vi "Set Z Voltage_test.vi"(2 "Z-Position":dbl) -> ()   [LabVIEW 2014]
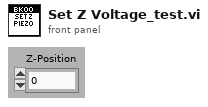
[diagram p1: front panel]
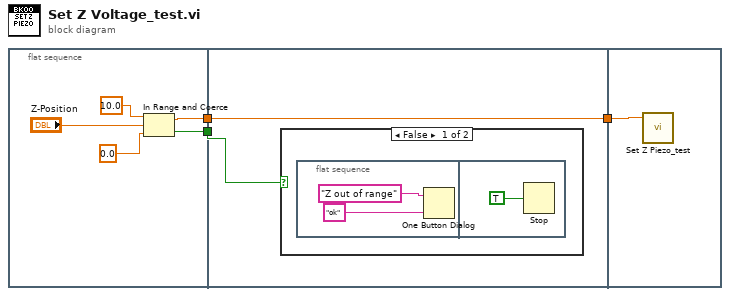
[diagram p0: block diagram]
diagram:
  n1 = flat-sequence {
    tunnel: [w5] -> w3
    tunnel: [w4] -> w1
    tunnel: w3 -> [w10]
    tunnel: [w10] -> w2
    tunnel: w1 -> [w9]
    tunnel: w2 -> [w14]
    frame #0 {
      n2 = In Range and Coerce(upper limit=10.0, x="Z-Position", lower limit=0.0) -> (coerced(x)=w5:dbl, In Range?=w4:bool)
    }
    frame #1 {
      n3 = case shown="False" w9 {
        frame False {
          n4 = flat-sequence {
            frame #0 {
              n5 = One Button Dialog(message="Z out of range", button name ("OK")="ok") -> ()  [unwired: 1 out]
            }
            frame #1 {
              n6 = Stop(stop? (T)=TRUE) -> ()
            }
          }
        }
        frame True {
        }
      }
    }
    frame #2 {
      n7 = call "Set Z Piezo_test.vi"("X Offset Voltage"=w14) -> ()  [unwired: 4 in]
    }
  }
